vi "IECal-Show Last N.vi"(0 "Expt State":T2, 5 "Mag graph":refnum<vi>, 7 "Phase graph":refnum<vi>, 9 "Speaker":T1, 11 "error in (no error)":errorcluster, 12 "Plot Max SPL":bool) -> (15 "error out":errorcluster)   [LabVIEW 2020]
doc: "This helper VI plots all of the in ear calibration files in the current experiment data folder.\n\nKEH 9/10/09"
uses:
  cfts/LV Source/CFTS Main Panel SubVIs/CFTS-Experiment State.ctl
  epl-vi-lib/Utility VIs/Type Defs/Speaker ring.ctl
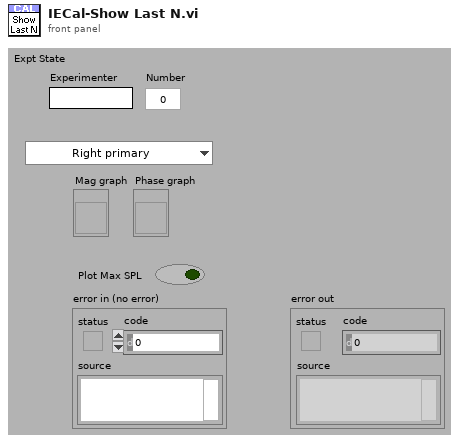
[diagram p1: front panel]
types:
  T1 = typedef "Speaker ring.ctl" = enum16{"Right primary", "Right secondary", "Left primary", "Left secondary"}
  T2 = typedef "CFTS-Experiment State.ctl" = cluster{"Experimenter":string, "Number":u32, "Right":string, "Left":string, "Data Folder":path, "State File":path, "Version Info":string, "End Exposure Time":dbl, "Exposure Duration":string, "Run #":cluster{"CAP":i16, "ABR":i16, "DP":i16, "VsEP":i16, "MeasSeq":i16, "SubSeq":i16, "SFOAE":i16}}
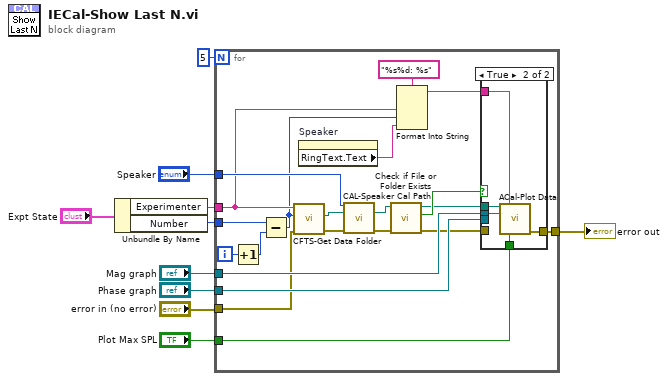
[diagram p0: block diagram]
diagram:
  n1 = Unbundle By Name("Expt State") -> ("Experimenter"=w2:string, "Number"=w1:u32)
  n2 = for {
    N: 5 -> [_]
    tunnel: "Mag graph" -> [w31]
    tunnel: "Phase graph" -> [w30]
    tunnel: "error in (no error)" -> [w17]
    tunnel: [w29] -> w10
    tunnel: "Plot Max SPL" -> [w26]
    tunnel: "Speaker" -> [w24]
    tunnel: w2 -> [w14]
    tunnel: w1 -> [w19]
    i -> [w20]
    n3 = Increment(x=w20) -> (x+1=w18:i32)
    n4 = Subtract(x=w19, y=w18) -> (x-y=w13:u32)
    n5 = call "CFTS-Get Data Folder.vi"("error in (no error)"=w17, "Number"=w13, "Experimenter"=w14) -> ("error out"=w21:errorcluster, "Data folder"=w25:path)  [unwired: 7 in]
    n6 = property on="Speaker" class="Enum (strict)"() -> ("RingText.Text"=w12:string)  [unwired: 2 in, 2 out]
    n7 = call "CAL-Speaker Cal Path.vi"("Speaker"=w24, "Data Folder"=w25, "error in (no error)"=w21) -> ("Cal Path"=w23:path, "error out"=w22:errorcluster)  [unwired: 11 in]
    n8 = call <vilib>:"Check if File or Folder Exists.vi"("error in (no error)"=w22, "path"=w23) -> ("error out"=w16:errorcluster, "file or folder exists?"=w28:bool, "dup path"=w27:path)  [unwired: 7 in]
    n9 = Format Into String(format string="%s%d: %s", w14, w13, w12) -> (resulting string=w11:string)  [unwired: 2 in, 1 out]
    n10 = case shown="True" w28 {
      tunnel: w31 -> [_ w35]
      tunnel: w30 -> [_ _]
      tunnel: w16 -> [w32 _]
      tunnel: [w32 w33] -> w29
      tunnel: w27 -> [_ w37]
      tunnel: w26 -> [_ w34]
      tunnel: w11 -> [_ w36]
      frame False {
      }
      frame True {
        n11 = call "ACal-Plot Data.vi"("Path"=w37, "Name"=w36, "Mag graph"=w35, "Plot max"=w34) -> ("error out"=w33:errorcluster)  [unwired: 10 in, 1 out]
      }
    }
  }
  "error out" <- w10
